vi "About_INL.vi"(8 "error in":errorcluster) -> (0 "error out":errorcluster)   [LabVIEW 2011]
uses:
  <vilib>/Platform/browser.llb/Open URL in Default Browser (string).vi
panel:
  in  "INL Weblink":bool
  # "INL repository maintained by: \nPieter De Beule & Marco Martins\nGPL license (www.gnu.org)"
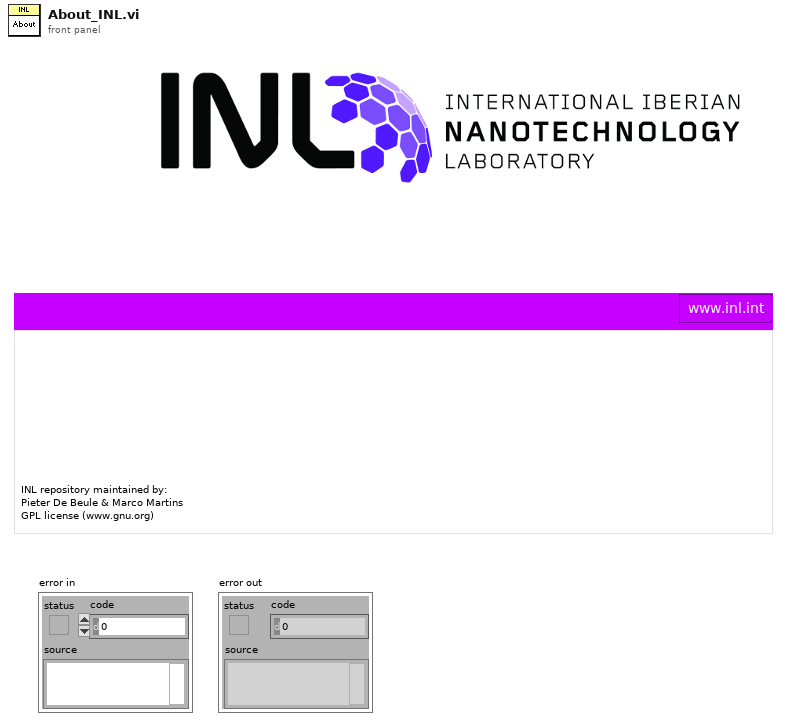
[diagram p1: front panel]
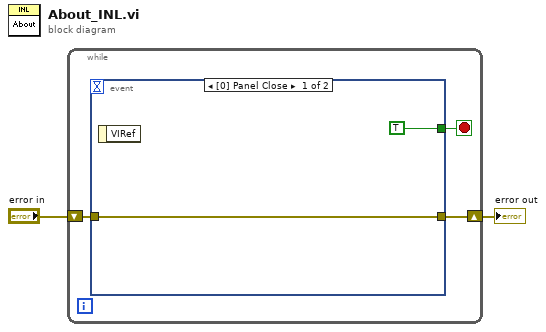
[diagram p0: block diagram]
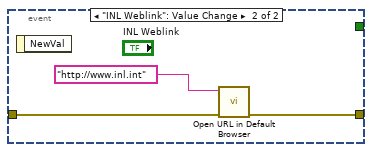
[diagram p2: hidden frame]
diagram:
  n1 = while {
    shift-right: [w4] -> w1
    shift-left: "error in" -> [w5]
    stop <- w3 stop-if-true
    n2 = event shown="[0] Panel Close" {
      selector: _ -> [_ _]
      dyn-events: _ -> [_ _]
      timeout: _ -> [_ _]
      tunnel: w5 -> [w7 w10]
      tunnel: [w7 w9] -> w4
      tunnel: [TRUE _] -> w3
      event Panel Close {
        n3 = event-data() -> ()  [unwired: 1 in, 1 out]
      }
      event "INL Weblink": Value Change {
        n4 = event-data() -> ()  [unwired: 1 in, 1 out]
        n5 = call-poly <vilib>:"Open URL in Default Browser.vi"("error in (no error)"=w10, "URL"="http://www.inl.int") -> ("error out"=w9:errorcluster)  [unwired: 4 in, 1 out]
      }
    }
  }
  "error out" <- w1
